vi "Trigger Generator FG.vi"(0 "Boolean in":bool) -> (1 "Falling Trigger out":bool, 2 "Rising Trigger out":bool)   [LabVIEW 2013]
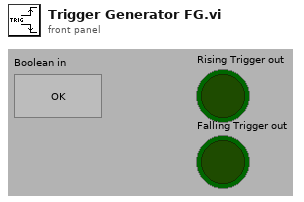
[diagram p1: front panel]
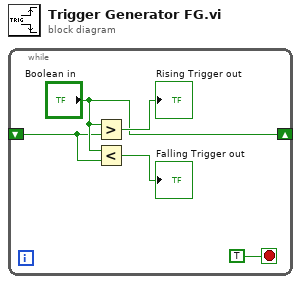
[diagram p0: block diagram]
diagram:
  n1 = while {
    shift-right: ["Boolean in"] -> _
    shift-left: _ -> [w2]
    stop <- TRUE stop-if-true
    n2 = Greater?(x="Boolean in", y=w2) -> (0:→"Rising Trigger out":bool)
    n3 = Less?(x="Boolean in", y=w2) -> (x < y?=→"Falling Trigger out":bool)
  }
